vi "local.Log In.vi"(0 "SLSC Local in":refnum<class "SLSC Local.lvclass">, 1 "username":string, 2 "password":string, 5 "chassis":refnum<k21>, 11 "error in (no error)":errorcluster, 12 "connect timeout (60 sec)":dbl=60.0, 13 "save credentials to disk? (F)":bool) -> (4 "SLSC Local out":refnum<class "SLSC Local.lvclass">, 15 "error out":errorcluster)   [LabVIEW 2016, in "SLSC Interfaces.lvlib" / "SLSC Local.lvclass"]
uses:
  SLSC Local.lvclass
  <vilib>/SLSC/SLSC.lvlib
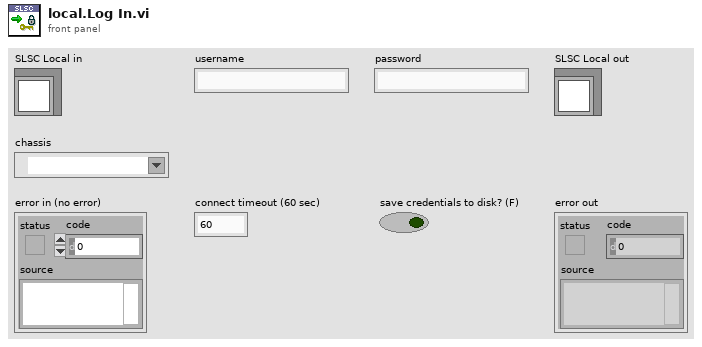
[diagram p1: front panel]
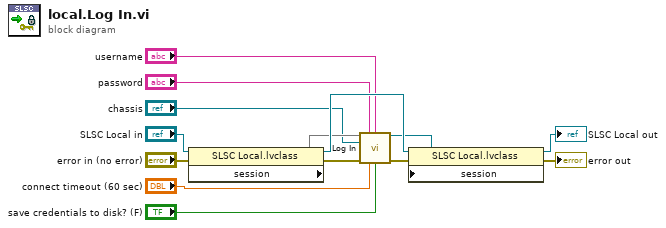
[diagram p0: block diagram]
diagram:
  n1 = property class="SLSC Local.lvclass"(reference="SLSC Local in", error in="error in (no error)") -> (reference out=w14:refnum<class "SLSC Local.lvclass">, error out=w8:errorcluster, "session"=w9)
  n2 = call <vilib>:"Log In.vi"("session in"=w9, "username"="password", "password"="username", "chassis"="chassis", "error in (no error)"=w8, "connect timeout (60 sec)"="connect timeout (60 sec)", "save credentials to disk? (F)"="save credentials to disk? (F)") -> ("session out"=w7:refnum<k21>, "error out"=w6:errorcluster)  [unwired: 7 in]
  n3 = property class="SLSC Local.lvclass"(reference=w14, error in=w6, "session"=w7) -> (reference out=→"SLSC Local out":refnum<class "SLSC Local.lvclass">, error out=→"error out":errorcluster)
